vi "create clear function.vi"(8 "error in (no error)":errorcluster) -> (0 "error out":errorcluster)   [LabVIEW 2010, in "TemplateGenerator.lvlib"]
uses:
  TemplateGenerator.lvlib
  Current Value Table.lvlib
  Type Defs/Memory Commands.ctl
  <vilib>/Utility/miscctls.llb/LVPointTypeDef.ctl
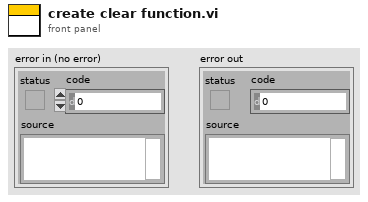
[diagram p1: front panel]
types:
  T1 = cluster{"VIPath":path, "Menu Name":string, "Selector Name":string}[]
  T2 = typedef "LVPointTypeDef.ctl" = cluster{"Horizontal":i16, "Vertical":i16}
  T3 = typedef "Current Value Table.lvlib/Memory Commands.ctl" = enum16{"Init", "Add Data", "Read", "Read Group", "Read All", "Write", "Write Group", "Get Size"}
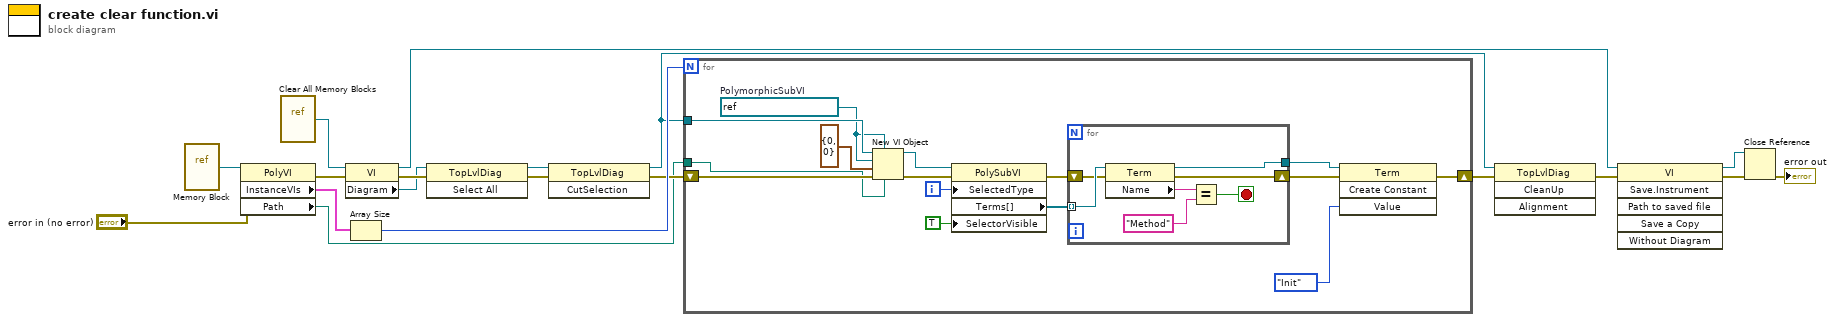
[diagram p0: block diagram]
diagram:
  n1 = vi-ref "Memory Block.vi"() -> (w6:refnum<vi>)
  n2 = property class="PolyVI"(reference=w6, error in="error in (no error)") -> (error out=w9:errorcluster, "InstanceVIs"=w16:T1, "Path"=w7:path)  [unwired: 1 out]
  n3 = vi-ref "Clear All Memory Blocks.vi"() -> (w1:refnum<vi>)
  n4 = property class="VI"(reference=w1, error in=w9) -> (reference out=w13:refnum<vi>, error out=w3:errorcluster, "Diagram"=w2:refnum<vi>)
  n5 = Array Size(array=w16) -> (size(s)=w17:i32)
  n6 = invoke class="TopLvlDiag" method="Select All"(reference=w2, error in=w3) -> (reference out=w5:refnum<vi>, error out=w4:errorcluster)  [unwired: 1 in, 1 out]
  n7 = invoke class="TopLvlDiag" method="CutSelection"(reference=w5, error in=w4) -> (reference out=w11:refnum<vi>, error out=w8:errorcluster)  [unwired: 1 in, 1 out]
  n8 = for {
    N: w17 -> [_]
    tunnel: w7 -> [w32]
    tunnel: w11 -> [w34]
    shift-right: [w21] -> w10
    shift-left: w8 -> [w33]
    i -> [w28]
    w31 = refnum<vi> refnum  # PolymorphicSubVI
    n9 = New VI Object(vi object class=w31, owner refnum=w34, style=w31, position/next to=T2 {"Horizontal"=0, "Vertical"=0} ("location"), 6:w32, 8:w33) -> (object refnum=w30:refnum<vi>, 0:w29:errorcluster)  [unwired: 2 in]
    n10 = property class="PolySubVI"(reference=w30, error in=w29, "SelectedType"=w28, "SelectorVisible"=TRUE ("Selector Visible")) -> (error out=w25:errorcluster, "Terms[]"=w26:refnum<vi>[])  [unwired: 1 out]
    n11 = for {
      tunnel: w26 -> [w41] mode=indexing
      shift-right: [w37] -> w24
      shift-left: w25 -> [w40]
      tunnel: [w35] -> w23
      stop <- w36 stop-if-true
      n12 = property class="Term"(reference=w41, error in=w40) -> (reference out=w35:refnum<vi>, error out=w37:errorcluster, "Name"=w39:string)
      n13 = Equal?(x=w39, y="Method") -> (x = y?=w36:bool)
    }
    n14 = invoke class="Term" method="Create Constant"(reference=w23, error in=w24, "Value"=Memory_Commands."Init" ("Method")) -> (error out=w21:errorcluster)  [unwired: 1 in, 3 out]
  }
  n15 = invoke class="TopLvlDiag" method="CleanUp"(reference=w11, error in=w10) -> (error out=w12:errorcluster)  [unwired: 2 in, 3 out]
  n16 = invoke class="VI" method="Save.Instrument"(reference=w13, error in=w12) -> (reference out=w15:refnum<vi>, error out=w14:errorcluster)  [unwired: 4 in, 4 out]
  n17 = Close Reference(reference=w15, error in (no error)=w14) -> (error out=→"error out":errorcluster)
